vi "PositionToReceivePass2ndStrikerDoublePass.vi"(6 "TimeElapsed?":bool=TRUE, 8 "error in (no error)":errorcluster, 9 "Game":refnum<class "Game.lvclass">, 10 "Robot":refnum<class "Robot.lvclass">, 11 "PositionToReceivePassSkill in":refnum<class "PositionToReceivePassSkill.lvclass">) -> (0 "error out":errorcluster, 2 "2ndStrikerPositionDoublePass":dbl[](array[numeric]), 3 "PositionToReceivePassSkill out":refnum<class "PositionToReceivePassSkill.lvclass">)   [LabVIEW 2023, in "PositionToReceivePassSkill.lvclass"]
uses:
  PositionToReceivePassSkill.lvclass
  Game_class/Game.lvclass
  Robot_class/Robot.lvclass
  Game_class/Game.lvclass/Game.ctl
  Parameters_class/Parameters.lvclass/Parameters.ctl
  Object_class/Object.lvclass/Object.ctl
  Game_class/Read Utilities.lvclass.vi
  Game_class/Read Parameters.lvclass.vi
  Game_class/Read FieldRef.vi
  Game_class/Read BallRef.vi
  Object_class/Read x.vi
  Object_class/Read y.vi
  Parameters_class/Read AttakingOurselves.vi
  Ball_class/Ball.lvclass
  C:/Users/roboi/Downloads/VSS_AI-Larc2023 - Copia (2)/Object_class/Object.lvclass
  Utilities_class/Utilities.lvclass
  Parameters_class/Parameters.lvclass
  Field_class/Field.lvclass
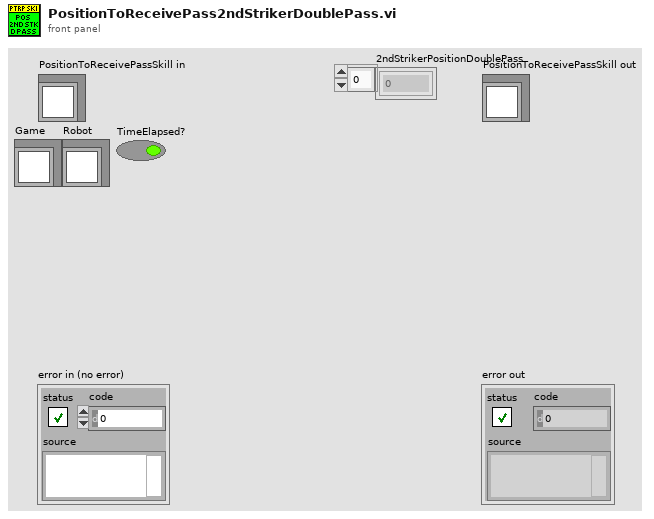
[diagram p1: front panel]
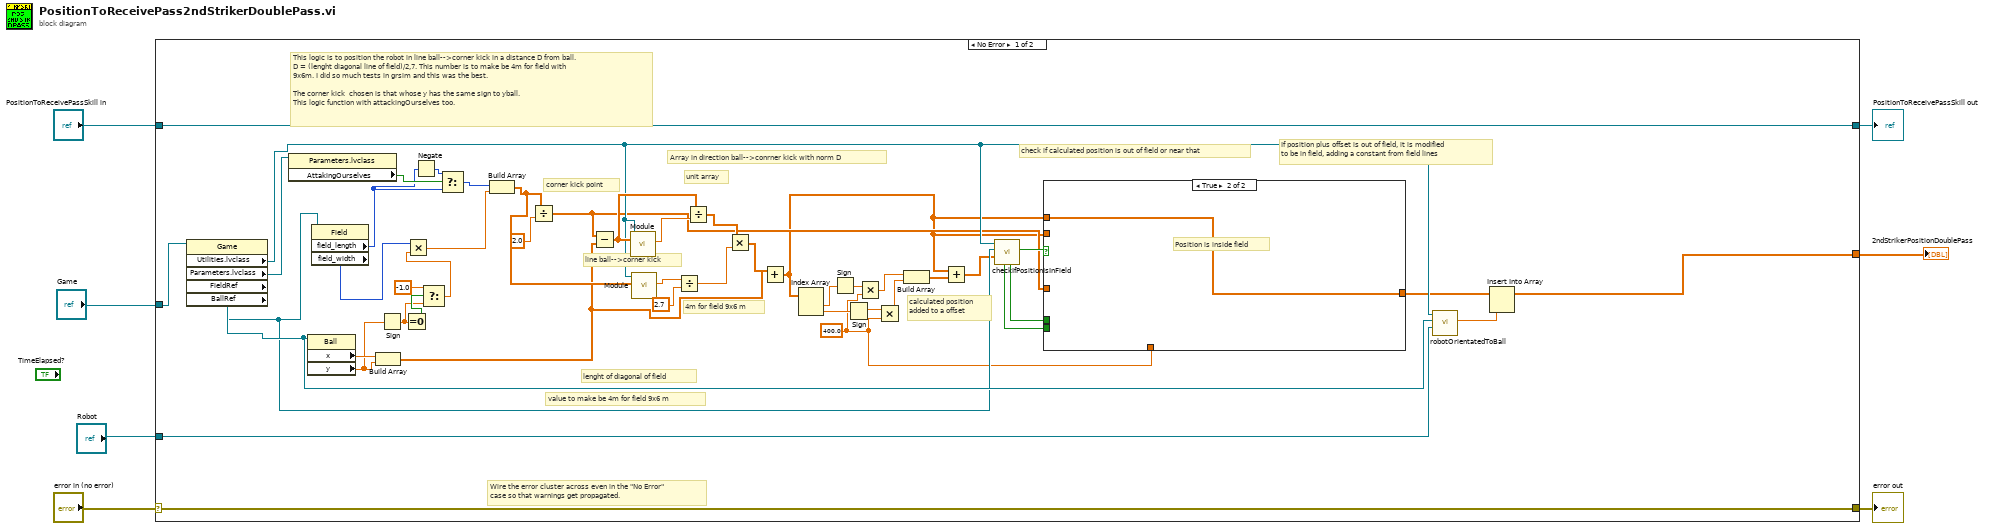
[diagram p0: block diagram]
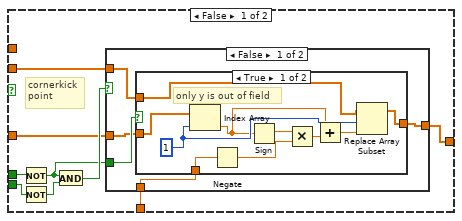
[diagram p2: hidden frame]
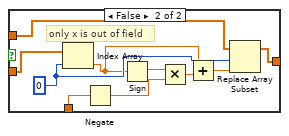
[diagram p3: hidden frame]
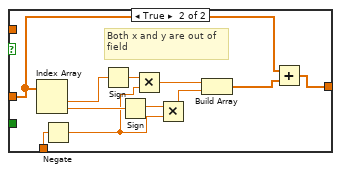
[diagram p4: hidden frame]
diagram:
  n1 = case shown="No Error" "error in (no error)" {
    selector: "error in (no error)" -> [w53 w102]
    tunnel: [w53 w102] -> w6
    tunnel: [w54 w101] -> w4
    tunnel: "PositionToReceivePassSkill in" -> [w54 w101]
    tunnel: "Game" -> [w21 _]
    tunnel: "Robot" -> [w32 _]
    tunnel: [w30 _] -> w1
    frame No Error {
      w14 = 400.0 ("y")
      # "If position plus offset is out of field, it is modified\nto be in field, adding a constant from field lines"
      # "calculated position\nadded to a offset"
      # "check if calculated position is out of field or near that"
      # "Array in direction ball-->conrner kick with norm D"
      # "This logic is to position the robot in line ball-->corner kick in a distance D from ball.\nD = (lenght diagonal line of field)/2,7. This number is to make be 4m for field with\n9x6m. I did so much tests in grsim and this was the best.\n\nThe corner kick  chosen is that whose y has the same sign to yball.\nThis logic function with attackingOurselves too."
      # "value to make be 4m for field 9x6 m"
      # "4m for field 9x6 m"
      # "lenght of diagonal of field"
      # "unit array"
      # "line ball-->corner kick"
      # "corner kick point"
      # "Wire the error cluster across even in the \"No Error\"\ncase so that warnings get propagated."
      n2 = property class="Game"(reference=w21) -> ("Utilities.lvclass"=w22:refnum<class "Utilities.lvclass">, "Parameters.lvclass"=w49:refnum<class "Parameters.lvclass">, "FieldRef"=w20:refnum<class "Field.lvclass">, "BallRef"=w31:refnum<class "Ball.lvclass">)  [unwired: 1 in, 2 out]
      n3 = property class="Parameters.lvclass"(reference=w49) -> ("AttakingOurselves"=w48:bool)  [unwired: 1 in, 2 out]
      n4 = property class="Ball"(reference=w31) -> ("x"=w52:dbl, "y"=w50:dbl)  [unwired: 1 in, 2 out]
      n5 = property class="Field"(reference=w20) -> ("field_length"=w46:i32, "field_width"=w51:i32)  [unwired: 1 in, 2 out]
      n6 = Build Array(w52, w50) -> (w34:dbl[])
      n7 = Sign(1:w50) -> (0:w10:dbl)
      n8 = Equal To 0?(x=w10) -> (x = 0?=w11:bool)
      n9 = Negate(x=w46) -> (-x=w47:i32)
      n10 = Select(t=-1.0, s=w11, f=w10) -> (s? t:f=w8:dbl)
      n11 = Multiply(x=w51, y=w8) -> (x*y=w44:dbl)
      n12 = Select(t=w47, s=w48, f=w46) -> (s? t:f=w45:i32)
      n13 = Build Array(w45, w44) -> (w39:dbl[])
      n14 = Divide(x=w39, y=2.0) -> (x/y=w15:dbl[])
      n15 = Subtract(x=w15, y=w34) -> (x-y=w42:dbl[])
      n16 = call "Module.vi"("2D vector"=w42, "Utilities in"=w22) -> ("Modulo"=w41:dbl)  [unwired: 7 in, 2 out]
      n17 = call "Module.vi"("2D vector"=w39, "Utilities in"=w22) -> ("Modulo"=w38:dbl)  [unwired: 7 in, 2 out]
      n18 = Divide(x=w38, y=2.7) -> (x/y=w36:dbl)
      n19 = Divide(x=w42, y=w41) -> (x/y=w40:dbl[])
      n20 = Multiply(x=w40, y=w36) -> (x*y=w35:dbl[])
      n21 = Add(x=w35, y=w34) -> (x+y=w13:dbl[])
      n22 = Index Array(array=w13) -> (element #1=w29:dbl, element #2=w26:dbl)  [unwired: 2 in]
      n23 = Sign(1:w29) -> (0:w28:dbl)
      n24 = Sign(1:w26) -> (0:w27:dbl)
      n25 = Multiply(x=w28, y=w14) -> (x*y=w25:dbl)
      n26 = Multiply(x=w27, y=w14) -> (x*y=w24:dbl)
      n27 = Build Array(w25, w24) -> (w23:dbl[])
      n28 = Add(x=w13, y=w23) -> (x+y=w12:dbl[])
      n29 = call "checkIfPositionIsInField.vi"("Position"=w12, "FieldRef"=w20, "Utilities in"=w22) -> ("Position Is In Field?"=w19:bool, "y Is in Field?"=w17:bool, "x Is in Field?"=w16:bool)  [unwired: 4 in, 2 out]
      n30 = case shown="True" w19 {
        tunnel: w13 -> [_ w100]
        tunnel: [w57 w100] -> w18
        tunnel: w17 -> [w62 _]
        tunnel: w16 -> [w61 _]
        tunnel: w15 -> [w59 _]
        tunnel: w14 -> [w58 _]
        tunnel: w13 -> [w55 _]
        frame False {
          # "cornerkick\npoint"
          n31 = Not(x=w62) -> (.not. x?=w56:bool)
          n32 = Not(x=w61) -> (.not. x?=w60:bool)
          n33 = And(x=w56, y=w60) -> (x .and. y?=w63:bool)
          n34 = case shown="False" w63 {
            tunnel: w59 -> [w64 w90]
            tunnel: w58 -> [w67 w92]
            tunnel: [w66 w89] -> w57
            tunnel: w56 -> [w68 _]
            tunnel: w55 -> [w65 _]
            frame False {
              n35 = case shown="True" w68 {
                tunnel: w65 -> [w69 w80]
                tunnel: w67 -> [w76 w86]
                tunnel: [w74 w84] -> w66
                tunnel: w64 -> [w70 w79]
                frame True {
                  w75 = 1
                  # "only y is out of field"
                  n36 = Index Array(array=w70, index=w75) -> (element=w71:dbl)
                  n37 = Negate(x=w76) -> (-x=w77:dbl)
                  n38 = Sign(1:w71) -> (0:w78:dbl)
                  n39 = Multiply(x=w78, y=w77) -> (x*y=w73:dbl)
                  n40 = Add(x=w71, y=w73) -> (x+y=w72:dbl)
                  n41 = Replace Array Subset(array=w69, new element=w72, index=w75) -> (w74:dbl[])
                }
                frame False {
                  w85 = 0
                  # "only x is out of field"
                  n42 = Index Array(array=w79, index=w85) -> (element=w81:dbl)
                  n43 = Negate(x=w86) -> (-x=w87:dbl)
                  n44 = Sign(1:w81) -> (0:w88:dbl)
                  n45 = Multiply(x=w88, y=w87) -> (x*y=w83:dbl)
                  n46 = Add(x=w81, y=w83) -> (x+y=w82:dbl)
                  n47 = Replace Array Subset(array=w80, new element=w82, index=w85) -> (w84:dbl[])
                }
              }
            }
            frame True {
              # "Both x and y are out of\nfield"
              n48 = Index Array(array=w90) -> (element #1=w99:dbl, element #2=w96:dbl)  [unwired: 2 in]
              n49 = Negate(x=w92) -> (-x=w93:dbl)
              n50 = Sign(1:w99) -> (0:w98:dbl)
              n51 = Sign(1:w96) -> (0:w97:dbl)
              n52 = Multiply(x=w98, y=w93) -> (x*y=w95:dbl)
              n53 = Multiply(x=w97, y=w93) -> (x*y=w94:dbl)
              n54 = Build Array(w95, w94) -> (w91:dbl[])
              n55 = Add(x=w90, y=w91) -> (x+y=w89:dbl[])
            }
          }
        }
        frame True {
          # "Position is inside field"
        }
      }
      n56 = call "robotOrientatedToBall.vi"("Robot"=w32, "BallRef"=w31, "Utilities in"=w22) -> ("Orientation"=w33:dbl)  [unwired: 6 in, 2 out]
      n57 = Insert Into Array(array=w18, new element=w33) -> (w30:dbl[])  [unwired: 1 in]
    }
    frame Error {
    }
  }
  "error out" <- w6
  "PositionToReceivePassSkill out" <- w4
  "2ndStrikerPositionDoublePass" <- w1
